vi "QuadEncTestHarness.vi"() -> ()   [LabVIEW 2015]
uses:
  QuadEnc/Parameters.ctl
  QuadEnc/Output.ctl
  <vilib>/Platform/TimedLoop/XDataNode/timing_clust.ctl
  <vilib>/Platform/TimedLoop/XDataNode/nitl_modes.ctl
  <vilib>/Platform/TimedLoop/XDataNode/wakeup.ctl
  <vilib>/rvi/Emulation/niFpgaSctlEmulationGetInTimedLoop.vi
  <vilib>/rvi/Emulation/niFpgaEmulationReportErrorSimple.vi
  <vilib>/rvi/Emulation/niFpgaGetClockAttributes.vi
  <vilib>/rvi/Emulation/niFpgaCriticalErrorInLSC.vi
  <vilib>/rvi/eio/common/nirviEmuTemplateMethod_errors.vi
  <vilib>/Platform/TimedLoop/XDataNode/XDataNode.xnode
  <vilib>/eio/EIONode/EIONode.xnode
  <vilib>/Platform/TimedLoop/XDataNode/XDNodeRunTimeDep.lvlib
  QuadEnc/QuadEnc.lvlib
panel:
  out "Output":T1
  out "CW_direction":bool
  out "RevPosition":i32
  out "AbsPosition":i32
  in  "reset":bool
  in  "Parameters":T2
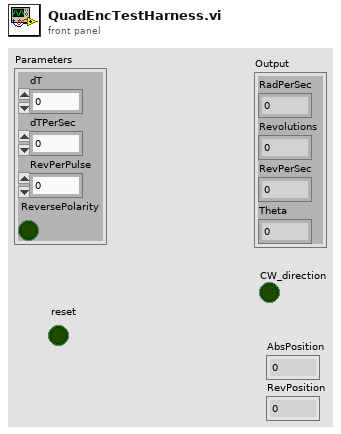
[diagram p1: front panel]
types:
  T1 = typedef "QuadEnc.lvlib/Output.ctl" = cluster{"RadPerSec":sgl, "Revolutions":sgl, "RevPerSec":sgl, "Theta":sgl}
  T2 = typedef "QuadEnc.lvlib/Parameters.ctl" = cluster{"dT":u32, "dTPerSec":sgl, "RevPerPulse":sgl, "ReversePolarity":bool}
  T3 = typedef "XDNodeRunTimeDep.lvlib/timing_clust.ctl" = cluster{"Expected End [f-1]":u64, "Actual End [f-1]":u64, "Finished Late? [f-1]":bool, "Expected End [i-1]":u64, "Actual End [i-1]":u64, "Finished Late? [i-1]":bool, "Expected Start [i]":u64, "Actual Start [i]":u64, "Expected Start [f]":u64, "Actual Start [f]":u64, "Source Name":string, "Structure Name":string, "Period":i64, "Deadline":i64, "Offset":i64, "Start":i64, "Priority":i32, "Timeout":i32, "Mode":T4, "Wakeup Reason":T5, "Error":errorcluster, "Source Type":string, "Secondary Source Type":string, "Global End Time":u64, "Global Start Time":u64, "Frame Duration":u64, "Iteration Duration":u64, "Assigned CPU":i32, "I/O Scan Engine Mode":u32}
  T4 = typedef "XDNodeRunTimeDep.lvlib/nitl_modes.ctl" = enum32{"No Change", "Process missed periods, maintain original phase", "Discard missed periods, maintain original phase", "Process missed periods, ignore original phase", "Discard missed periods, ignore original phase"}
  T5 = typedef "XDNodeRunTimeDep.lvlib/wakeup.ctl" = enum32{"Normal", "Aborted", "Asynchronous wakeup", "Timing source error", "Timed loop error", "Timeout"}
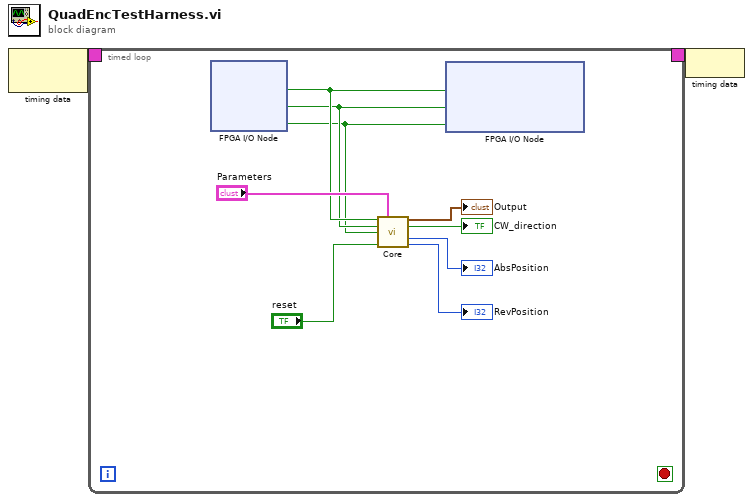
[diagram p0: block diagram]
diagram:
  n1 = node-c288() -> (w2:T3)  [unwired: 1 in]
  n2 = timed-loop {
    timing: w2 -> [_]
    timing-out: [_] -> w1
    stop <- _ stop-if-true
    n3 = xnode "FPGA I/O Node"() -> ("Enc_A"=w10:bool, "Enc_B"=w9:bool, "Enc_Z"=w8:bool)  [unwired: 3 in, 3 out]
    n4 = call "Core.vi"("A"=w10, "Parameters"="Parameters", "B"=w9, "Z"=w8, "reset"="reset") -> ("Output"=→"Output":T1, "CW_direction"=→"CW_direction":bool, "AbsPosition"=→"AbsPosition":i32, "RevPosition"=→"RevPosition":i32)  [unwired: 7 in]
    n5 = xnode "FPGA I/O Node"("GPIC/LVTTL/DIO3"=w10, "GPIC/LVTTL/DIO4"=w9, "GPIC/LVTTL/DIO5"=w8) -> ()  [unwired: 3 in, 3 out]
  }
  n6 = node-c288(w1) -> ()
